vi "ProdaNG.ProductionLines.Get.vi"(8 "error in (no error)":errorcluster, 11 "dbHandleIn":i32) -> (0 "error out":errorcluster, 2 "ProdLines":T1[](array[typedef]), 3 "dbHandle":i32)   [LabVIEW 2016]
doc: "This function returns a product structure for a product, which is identified by a part and a serial number.\nImportant information: The field 'individual' was taken over from the field 'allgemein' of the legacy data directly. Because of this most products have the value 0 further on and only a few the value 1. \nParameter:\nhandle is an Integer, which is returned by the function Login() at the creation of a new connection.\nwabcoPartId is the Id of the part.\nserialNumber is the serial number of the product for the part above.\nproduct is a pointer on a product structure, which is filled if the returncode is 0. The structure must be defined in the calling program.\n\nReturncodes:\n0 No error\n< 0 ORACLE Error code\n6 (ERROR_INVALID_HANDLE) in case of an invalid handle\n1403 Record does not exist"
uses:
  Controls/ProdaNG.ProdutionLine.ctl
  Controls/ProdaNG.ProductionLineSize.ctl
  <vilib>/Utility/importsl/GetValueByPointer/datatype.ctl
  <vilib>/Utility/importsl/GetValueByPointer/GetValueByPointer.xnode
  prodllNG.dll
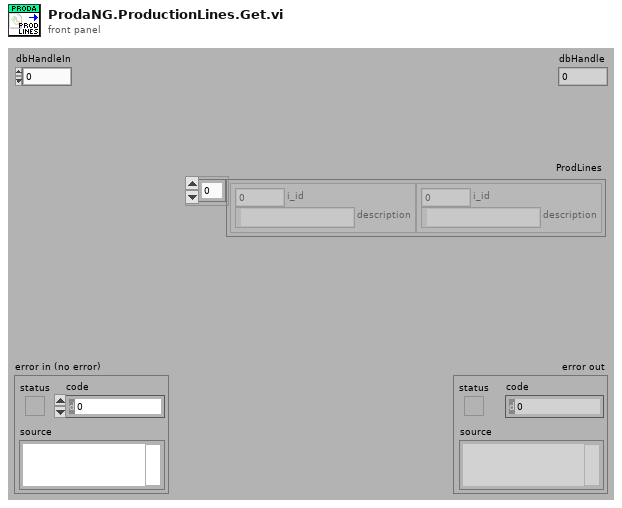
[diagram p1: front panel]
types:
  T1 = typedef "ProdaNG.ProdutionLine.ctl" = cluster{"i_id":i32, "description":string}
  T2 = typedef "ProdaNG.ProductionLineSize.ctl" = cluster{"product_wabcoNumber":i32, "product_serialNumber":i32, "component_wabcoNumber":i32, "component_serialNumber":i32, "pressStepResultId":i32, "qty":i32, "level":i32}
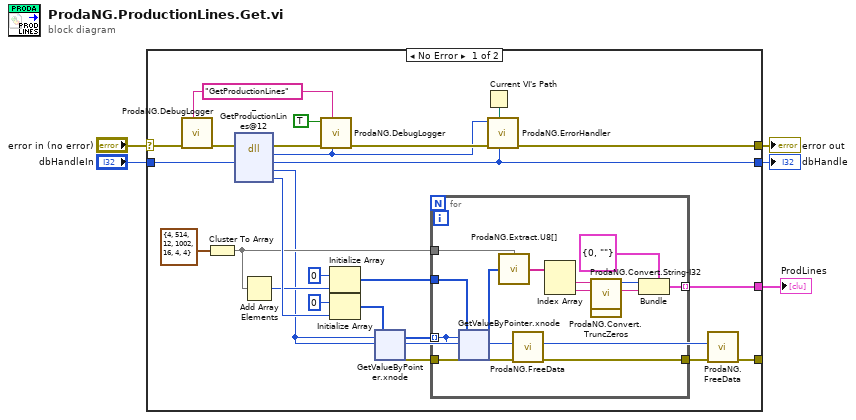
[diagram p0: block diagram]
diagram:
  n1 = case shown="No Error" "error in (no error)" {
    selector: "error in (no error)" -> [w25 w76]
    tunnel: [w30 w76] -> w4
    tunnel: "dbHandleIn" -> [w27 w75]
    tunnel: [w28 w75] -> w2
    tunnel: [w10 _] -> w1
    tunnel: [w7 _] -> _
    frame No Error {
      w21 = "GetProductionLines" ("cmd")
      n2 = call "ProdaNG.DebugLogger.vi"("cmd"=w21, "error in (no error)"=w25) -> ("error out"=w24:errorcluster)  [unwired: 9 in]
      n3 = Cluster To Array(cluster=T2 {"product_wabcoNumber"=4, "product_serialNumber"=514, "component_wabcoNumber"=12, "component_serialNumber"=1002, "pressStepResultId"=16, "qty"=4, "level"=4} ("ProductionLineSize")) -> (array=w11:i32[])
      n4 = dll-call lib="D:/svn/LineTraceSystem/SOFTWARE/sources/Database/ProdaNG/prodllNG.dll" fn="_GetProductionLines@12" ("ProDLL wrapper.dll:ProDLL_wrapper_GetWabcoParts_GetData")(error in=w24, "dbHandle"=w27) -> (error out=w23:errorcluster, "return type"=w20:i32, "dbHandle"=w28:i32, "prodLinesPtr"=w8:u32, "countPtr"=w15:i32)  [unwired: 4 in, 1 out]
      n5 = Add Array Elements(numeric array=w11) -> (sum=w12:i32)
      n6 = call "ProdaNG.DebugLogger.vi"("return type"=w20, "cmd"=w21, "error in (no error)"=w23, "done? (F)"=TRUE) -> ("error out"=w22:errorcluster)  [unwired: 7 in]
      n7 = Initialize Array(u8 0 ("element"), w12) -> (w13:u8[])
      n8 = Initialize Array(u32 0 ("element"), w15) -> (w19:u32[])
      n9 = xnode "GetValueByPointer.xnode"("Pointer"=w8, "InputType"=w19) -> ("Output"=w16:u32[], "ErrorOut"=w17:errorcluster)  [unwired: 2 in]
      n10 = for {
        tunnel: w17 -> [w44]
        tunnel: w16 -> [w36] mode=indexing
        tunnel: w13 -> [w43]
        tunnel: w11 -> [w38]
        tunnel: [w37] -> w10 mode=indexing
        tunnel: [w34] -> w9
        n11 = xnode "GetValueByPointer.xnode"("Pointer"=w36, "InputType"=w43, "ErrorIn"=w44) -> ("Output"=w40:u8[], "ErrorOut"=w35:errorcluster)  [unwired: 1 in]
        n12 = call "ProdaNG.Extract.U8[].vi"("unsigned byte array"=w40, "Sizes"=w38) -> ("Elements"=w39:string[])
        n13 = call "ProdaNG.FreeData.vi"("error in (no error)"=w35, "Pointers"=w36) -> ("error out"=w34:errorcluster)  [unwired: 9 in]
        n14 = Index Array(array=w39) -> (element #1=w41:string, element #2=w32:string)  [unwired: 2 in]
        n15 = call "ProdaNG.Convert.String-I32.vi"("unsigned byte string"=w41) -> ("32bit integer"=w42:i32)  [unwired: 10 in]
        n16 = call "ProdaNG.Convert.TruncZeros.vi"("string with \\0s"=w32) -> ("LV string"=w31:string)  [unwired: 10 in]
        n17 = Bundle(cluster=T1 {"i_id"=0, "description"=""} ("ProcessStep"), "i_id"=w42, "description"=w31) -> (w37:T1)
      }
      n18 = Current VI's Path() -> (path=w29:path)
      n19 = call "ProdaNG.ErrorHandler.vi"("dbHandleIn"=w28, "Path"=w29, "error in"=w22, "output_parameter"=w20) -> ("error out"=w30:errorcluster)  [unwired: 7 in]
      n20 = call "ProdaNG.FreeData.vi"("error in (no error)"=w9, "Pointers"=w8) -> ("error out"=w7:errorcluster)  [unwired: 9 in]
    }
    frame Error {
    }
  }
  "error out" <- w4
  "dbHandle" <- w2
  "ProdLines" <- w1
